vi "practica113c.vi"() -> ()   [LabVIEW 2013]
uses:
  <vilib>/Native 3D Graph/xcontrol/3DPC_SurfacePlot.xctl
panel:
  in  "stop":bool
  in  "s2":dbl
  in  "s1":dbl
  out "3D Graph":refnum<class "Base Datatype.lvclass">[](xcontrol)
  in  "xy 2":dbl(knob) scale=-175.0..175.0
  in  "yz":dbl(knob) scale=0.0..360.0
  in  "xy":dbl(knob) scale=0.0..360.0
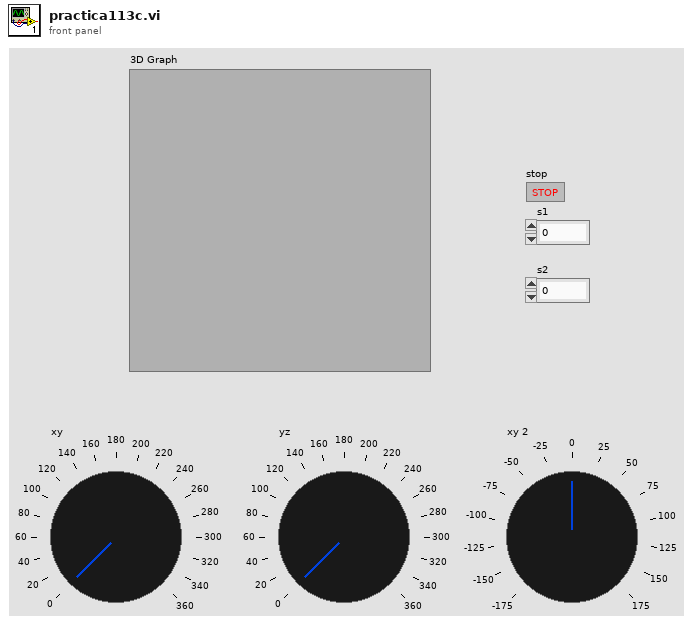
[diagram p1: front panel]
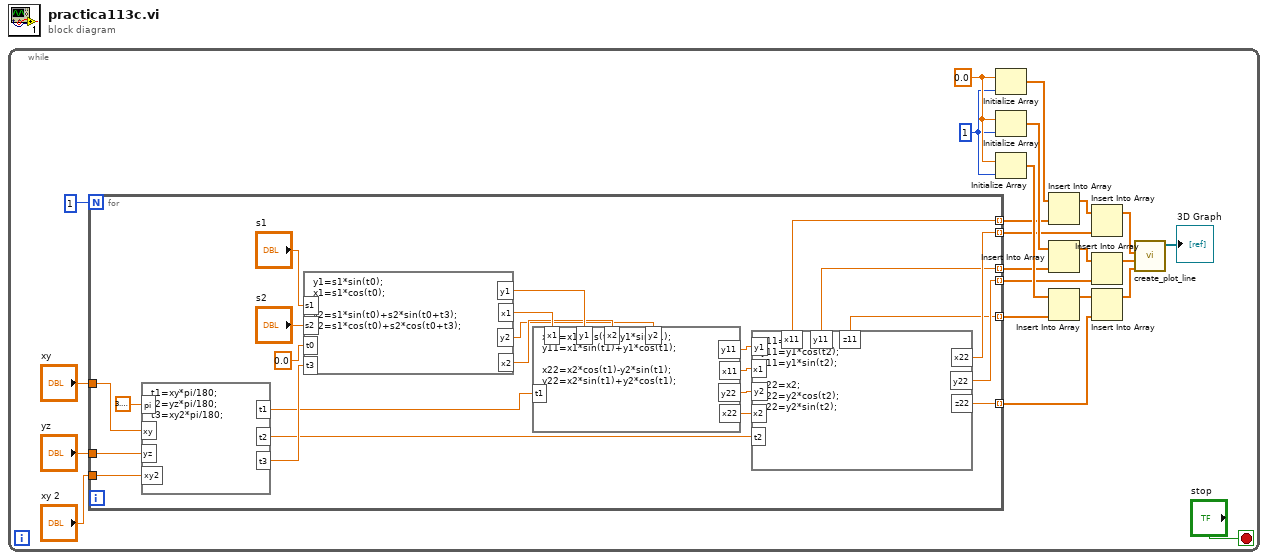
[diagram p0: block diagram]
diagram:
  n1 = while {
    stop <- "stop" stop-if-true
    w8 = 0.0
    w5 = 1 ("dimension size")
    n2 = for {
      N: 1 -> [_]
      tunnel: "xy" -> [w46]
      tunnel: "yz" -> [w45]
      tunnel: "xy 2" -> [w44]
      tunnel: [w29] -> w7 mode=indexing
      tunnel: [w28] -> w6 mode=indexing
      tunnel: [w27] -> w4 mode=indexing
      tunnel: [w26] -> w3 mode=indexing
      tunnel: [w25] -> w2 mode=indexing
      tunnel: [w24] -> w1 mode=indexing
      n3 = formula code="t1=xy*pi/180;\nt2=yz*pi/180;\nt3=xy2*pi/180;"("pi"=3.141592653589793, "xy"=w46, "yz"=w45, "xy2"=w44) -> ("t1"=w37:dbl, "t2"=w30:dbl, "t3"=w42:dbl)
      n4 = formula code="y1=s1*sin(t0);\nx1=s1*cos(t0);\n\ny2=s1*sin(t0)+s2*sin(t0+t3);\nx2=s1*cos(t0)+s2*cos(t0+t3);"("t0"=0.0 ("input variable"), "s1"="s1", "s2"="s2", "t3"=w42) -> ("y1"=w38:dbl, "x1"=w39:dbl, "y2"=w35:dbl, "x2"=w36:dbl)
      n5 = formula code="x11=x1*cos(t1)-y1*sin(t1);\ny11=x1*sin(t1)+y1*cos(t1);\n\nx22=x2*cos(t1)-y2*sin(t1);\ny22=x2*sin(t1)+y2*cos(t1);"("x1"=w39, "y1"=w38, "t1"=w37, "x2"=w36, "y2"=w35) -> ("y11"=w34:dbl, "x11"=w33:dbl, "y22"=w32:dbl, "x22"=w31:dbl)
      n6 = formula code="x11=x1;\ny11=y1*cos(t2);\nz11=y1*sin(t2);\n\nx22=x2;\ny22=y2*cos(t2);\nz22=y2*sin(t2);"("y1"=w34, "x1"=w33, "y2"=w32, "x2"=w31, "t2"=w30) -> ("x11"=w28:dbl, "y11"=w26:dbl, "z11"=w25:dbl, "x22"=w29:dbl, "y22"=w27:dbl, "z22"=w24:dbl)
    }
    n7 = Initialize Array(w8, w5) -> (w15:dbl[])
    n8 = Initialize Array(w8, w5) -> (w16:dbl[])
    n9 = Initialize Array(w8, w5) -> (w17:dbl[])
    n10 = Insert Into Array(array=w15, new element=w6) -> (w12:dbl[])  [unwired: 1 in]
    n11 = Insert Into Array(array=w16, new element=w3) -> (w13:dbl[])  [unwired: 1 in]
    n12 = Insert Into Array(array=w17, new element=w2) -> (w14:dbl[])  [unwired: 1 in]
    n13 = Insert Into Array(array=w12, new element=w7) -> (w9:dbl[])  [unwired: 1 in]
    n14 = Insert Into Array(array=w13, new element=w4) -> (w10:dbl[])  [unwired: 1 in]
    n15 = Insert Into Array(array=w14, new element=w1) -> (w11:dbl[])  [unwired: 1 in]
    n16 = call <vilib>:"create_plot_line.vi"("z vector"=w11, "y vector"=w10, "x vector"=w9) -> ("plots out"=→"3D Graph":refnum<class "Base Datatype.lvclass">[])  [unwired: 2 in, 6 out]
  }
